vi "ReturnFrame.vi"(8 "error in (no error)":errorcluster, 9 "block":u32=1, 10 "sample":u32=1, 11 "camera":u16=1) -> (0 "error out":errorcluster, 1 "Data Values Out 2":u16[](graph), 2 "Data Values Out 1":u16[](graph))   [LabVIEW 2015, in "ESLSCDLL.lvlib"]
uses:
  ESLSCDLL.lvlib
  Globals.vi
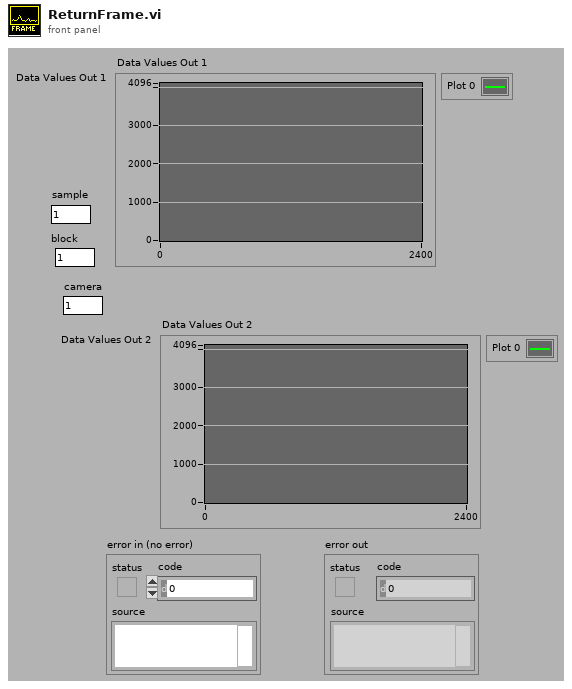
[diagram p1: front panel]
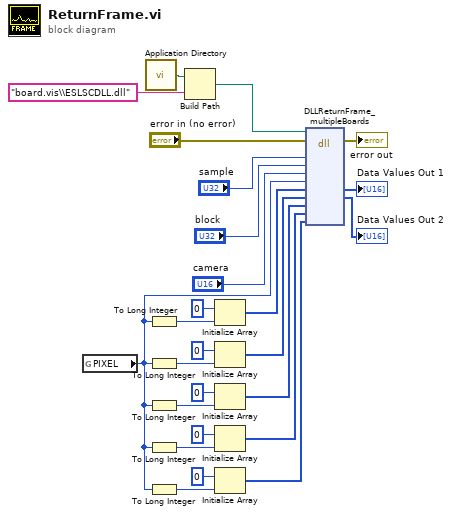
[diagram p0: block diagram]
diagram:
  n1 = global read "Globals.vi" "PIXEL"() -> (w4:u32)
  n2 = call <vilib>:"Application Directory.vi"() -> ("Application Directory"=w15:path)
  n3 = To Long Integer(number=w4) -> (32bit integer=w21:i32)
  n4 = To Long Integer(number=w4) -> (32bit integer=w18:i32)
  n5 = To Long Integer(number=w4) -> (32bit integer=w9:i32)
  n6 = To Long Integer(number=w4) -> (32bit integer=w7:i32)
  n7 = To Long Integer(number=w4) -> (32bit integer=w5:i32)
  n8 = Build Path(base path=w15, name or relative path="board.vis\\ESLSCDLL.dll") -> (appended path=w13:path)
  n9 = Initialize Array(u16 0, w21) -> (w20:u16[])
  n10 = Initialize Array(u16 0, w18) -> (w11:u16[])
  n11 = Initialize Array(u16 0, w9) -> (w3:u16[])
  n12 = Initialize Array(u16 0, w7) -> (w2:u16[])
  n13 = Initialize Array(u16 0, w5) -> (w1:u16[])
  n14 = dll-call lib="C:/ENTW/PCIE/LV64/board.vis/ESLSCDLL.dll" fn="DLLReturnFrame_multipleBoards" ("lwlscdll.dll:DLLReadFFLoop")(path in=w13, error in="error in (no error)", "sample"="sample", "block"="block", "camera"="camera", "pixel"=w4, "pdest0"=w20, "pdest1"=w11, "pdest2"=w3, "pdest3"=w2, "pdest4"=w1) -> (error out=→"error out":errorcluster, "pdest0"=→"Data Values Out 1":u16[], "pdest1"=→"Data Values Out 2":u16[])  [unwired: 9 in, 1 out]
